vi "建立局部变量.vi"() -> ()   [LabVIEW 2010]
panel:
  out "系统启动":bool
  in  "操作者姓名":string
  in  "流量":dbl format="%.2f"
  in  "压力":dbl format="%.2f"
  in  "温度":dbl format="%.2f"
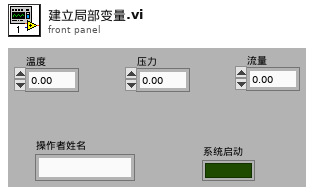
[diagram p1: front panel]
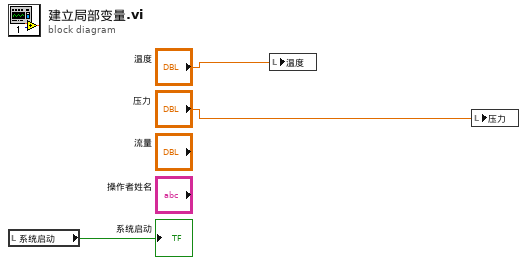
[diagram p0: block diagram]
diagram:
  n1 = local read "系统启动"() -> (→"系统启动":bool)
  n2 = local write "温度"("温度") -> ()
  n3 = local write "压力"("压力") -> ()
